vi "Configure AC Voltage Filter.vi"(8 "error in (no error)":errorcluster, 10 "AC Voltage Filter Type (0: Fast)":enum16{"Fast", "Middle", "Slow"}(ring), 11 "VISA resource name":refnum<visa-resource-name>) -> (0 "error out":errorcluster, 3 "VISA resource name out":refnum<visa-resource-name>)   [LabVIEW 2020, in "Library Instrument & Equipement.lvlib" / "Library Multimeter.lvlib" / "RIGOL DM3058.lvlib"]
doc: "Configures the AC Voltage Filter. \n\n<B>Note:</B>\n(1) This VI only applies to RIGOL DM3051 model.\n\n(2) This VI only available when setting the <B>Function</B> to AC Volts in <B>Configure Measurement.vi</B>."
uses:
  RIGOL DM3058.lvlib
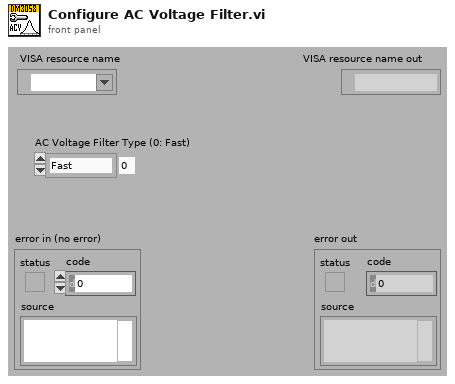
[diagram p1: front panel]
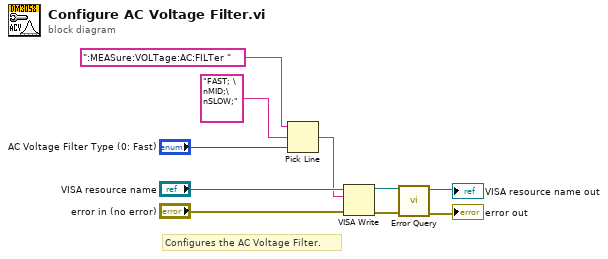
[diagram p0: block diagram]
diagram:
  # "Configures the AC Voltage Filter."
  n1 = Pick Line(string ("")=":MEASure:VOLTage:AC:FILTer ", multi-line string="FAST; \nMID;\nSLOW;", line index="AC Voltage Filter Type (0: Fast)") -> (output string=w9:string)
  n2 = VISA Write(VISA resource name="VISA resource name", write buffer=w9, error in (no error)="error in (no error)") -> (VISA resource name out=w4:refnum<visa-resource-name>, error out=w3:errorcluster)  [unwired: 1 out]
  n3 = call "Error Query.vi"("error in (no error)"=w3, "VISA resource name"=w4) -> ("error out"=→"error out":errorcluster, "VISA resource name out"=→"VISA resource name out":refnum<visa-resource-name>)  [unwired: 6 in, 2 out]
